vi "Check Current Trigger Level.vi"(8 "error in (no error)":errorcluster, 11 "VISA resource name":refnum<visa-resource-name>) -> (0 "error out":errorcluster, 2 "Current Trigger Level":dbl, 3 "VISA resource name out":refnum<visa-resource-name>)   [LabVIEW 2022 SP3, in "MagnaDC.lvlib"]
uses:
  MagnaDC.lvlib
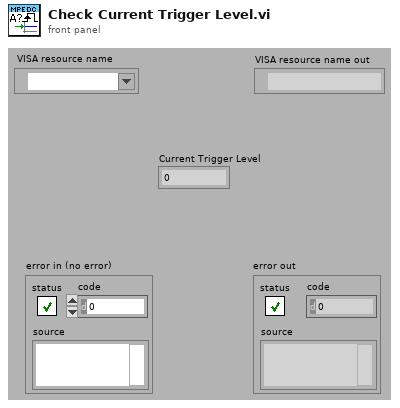
[diagram p1: front panel]
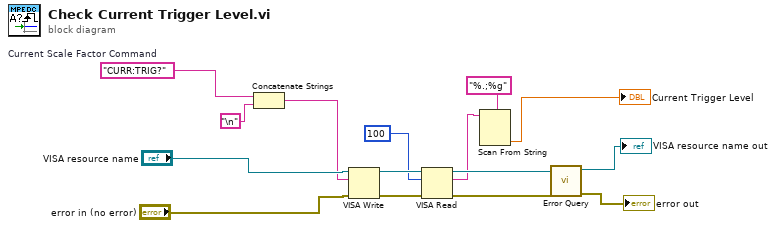
[diagram p0: block diagram]
diagram:
  w15 = "CURR:TRIG?"  # Current Scale Factor Command
  n1 = Concatenate Strings(w15, "\n") -> (w11:string)
  n2 = VISA Write(VISA resource name="VISA resource name", write buffer=w11, error in (no error)="error in (no error)") -> (VISA resource name out=w9:refnum<visa-resource-name>, error out=w10:errorcluster)  [unwired: 1 out]
  n3 = VISA Read(VISA resource name=w9, byte count=u32 100, error in (no error)=w10) -> (VISA resource name out=w7:refnum<visa-resource-name>, read buffer=w1:string, error out=w6:errorcluster)  [unwired: 1 out]
  n4 = Scan From String(format string="%.;%g", input string=w1) -> (output 1=→"Current Trigger Level":dbl)  [unwired: 3 in, 3 out]
  n5 = call "Error Query.vi"("error in (no error)"=w6, "VISA resource name"=w7) -> ("error out"=→"error out":errorcluster, "VISA resource name out"=→"VISA resource name out":refnum<visa-resource-name>)  [unwired: 6 in, 2 out]
